vi "MM6.InitSpecDevs.vi"(0 "i ref in":refnum<vi>, 2 "InitObjs":string[](array[string]), 3 "ms timeout (10000)":i32=10000, 5 "error in (no error)":errorcluster) -> (14 "i ref out":refnum<vi>, 16 "InitObjs out":string[](array[string]), 17 "timed out":bool, 19 "error out":errorcluster)   [LabVIEW 2014, in "MM6.lvlib"]
doc: "Initializes the special devices"
uses:
  MM6.lvlib
  CS_Core/BaseProcess/BaseProcess.lvlib
  LEBITLib/LEBITLib.lvlib
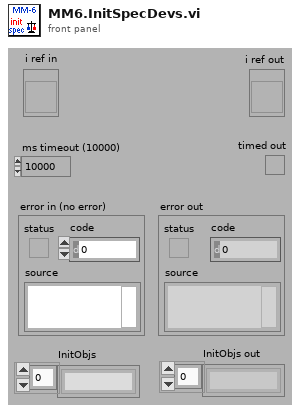
[diagram p1: front panel]
types:
  T1 = enum16{"simple", "synchronous", "asynchronous", "notification"}
  T2 = typedef "MM6.lvlib/MM6.i attribute.ctl" = cluster{"ConfigData":T3, "UsedObjs":string[], "ActScanStep":i32[], "AbortRequest":bool, "StopRequest":bool, "# cycles":i32, "Connected":bool, "MMStatus":T18, "# data":i32, "DIMServices":cluster{"MM6StatusString":string, "MM6StatusID":i32, "discArchiver":string, "discArchiverID":i32, "eventBuilder":string, "eventBuilderID":i32, "GUIIDString":string, "GUIIDStringID":i32}, "dataFile":string, "ExtraDataSets":T19, "PGRunning":T20}
  T3 = typedef "LEBITDefs.lvlib/LEBITDefs.ConfigData.ctl" = cluster{"GenConfig":T4, "Configs":T6[]}
  T4 = typedef "LEBITDefs.lvlib/LEBITDefs.GenConfig.ctl" = cluster{"Mode":i32, "Logs":T5[]}
  T5 = typedef "LEBITDefs.lvlib/LEBITDefs.Log.ctl" = cluster{"Name":string, "FctName":string, "Special":string}
  T6 = typedef "LEBITDefs.lvlib/LEBITDefs.OneConfig.ctl" = cluster{"MCA":T7, "Timing":T8, "Scans":T11[], "FreqDevs":T12[], "CleanDev":T13, "NrCycles":i32, "Specials":T15[], "Delays":T16[], "DAC":T17}
  T7 = typedef "LEBITDefs.lvlib/LEBITDefs.MCA.ctl" = cluster{"Name":string, "Address":string, "NrChannels":i32, "Gate":i32, "NrPipse":i32}
  T8 = typedef "LEBITDefs.lvlib/LEBITDefs.Timing.ctl" = cluster{"TimeTables":cluster{"TimeTable":T9}[], "Memories":T10[], "ScanX":string, "ScanY":string}
  T9 = typedef "LEBITDefs.lvlib/LEBITDefs.Timetable.ctl" = dbl[]
  T10 = typedef "LEBITDefs.lvlib/LEBITDefs.Memory.ctl" = cluster{"Device":string, "ExtTrig":bool, "TT2Use":i32, "PatternTable":string[]}
  T11 = typedef "LEBITDefs.lvlib/LEBITDefs.ScanDev.ctl" = cluster{"Name":string, "FctName":string, "Values":dbl[], "NrScanVals":i32, "Special":string}
  T12 = typedef "LEBITDefs.lvlib/LEBITDefs.FreqDev.ctl" = cluster{"Name":string, "Amp":dbl, "CenterFreq":dbl, "Time":dbl}
  T13 = typedef "LEBITDefs.lvlib/LEBITDefs.CleanDev.ctl" = cluster{"Name":string, "CleanData":T14[]}
  T14 = typedef "LEBITDefs.lvlib/LEBITDefs.CleanDataType.ctl" = cluster{"Amp":dbl, "Center":dbl, "Plus":dbl, "Minus":dbl, "Time":dbl}
  T15 = typedef "LEBITDefs.lvlib/LEBITDefs.Special.ctl" = cluster{"Name":string, "FctName":string, "VerySpecial":string, "Data":dbl}
  T16 = typedef "LEBITDefs.lvlib/LEBITDefs.Delay.ctl" = cluster{"Name":string, "Delay":dbl}
  T17 = typedef "LEBITDefs.lvlib/LEBITDefs.DAC.ctl" = cluster{"Name":string, "Step1":i32, "Step2":i32}
  T18 = typedef "MM6.lvlib/MM6.status.ctl" = enum16{"loaded", "load_error", "config", "config_error", "init", "init_error", "data_reset", "data_reset_error", "running", "start_error", "run_error", "abort_requested", "aborted", "stop_requested", "stopped", "stop_error", "Connected", "NOTConnected"}
  T19 = typedef "LEBITDefs.lvlib/LEBITDefs.ExtraData.ctl" = cluster{"Ions":cluster{"ExcitIonMass":string, "ExcitIonCharge":i32, "CleanIons":cluster{"CleanIonMass":string, "CleanIonCharge":i32}[]}, "TimingDescription":cluster{"TimeTableDescription":cluster{"Times":string[]}[], "PatternTableDescription":cluster{"Pattern":string[]}[]}, "ScanUnits":string[]}[]
  T20 = typedef "PPG_ABC.lvlib/PPG_ABC.PG_Running.ctl" = i32
  T21 = typedef "CoreDefs.rawDataType.ctl" = i8[]
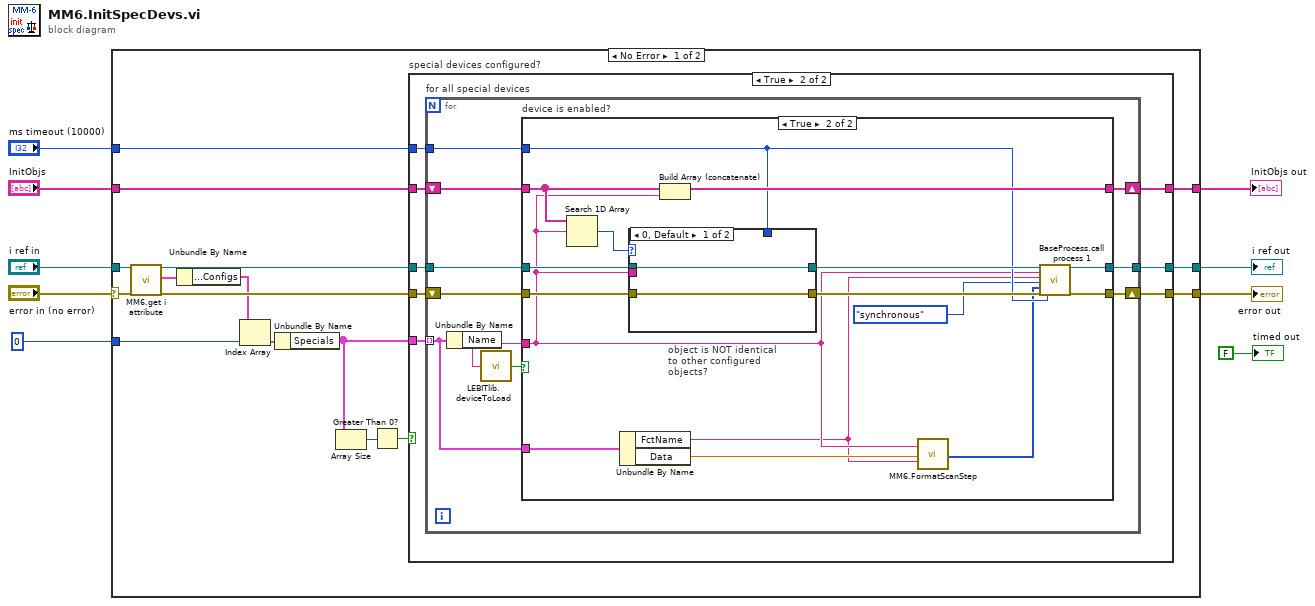
[diagram p0: block diagram]
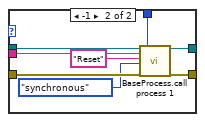
[diagram p4: hidden frame]
diagram:
  n1 = case shown="No Error" "error in (no error)" {
    selector: "error in (no error)" -> [w17 w76]
    tunnel: "i ref in" -> [w22 w77]
    tunnel: [w21 w77] -> w8
    tunnel: [w20 w76] -> w7
    tunnel: "InitObjs" -> [w19 w78]
    tunnel: [w18 w78] -> w4
    tunnel: 0 ("index") -> [w12 _]
    tunnel: "ms timeout (10000)" -> [w10 _]
    frame No Error {
      n2 = call "MM6.get i attribute.vi"("i ref in"=w22, "error in (no error)"=w17) -> ("i ref out"=w24:refnum<vi>, "i attribute"=w14:T2, "error out"=w23:errorcluster)  [unwired: 15 in]
      n3 = Unbundle By Name(w14) -> ("ConfigData.Configs"=w13:T6[])
      n4 = Index Array(array=w13, index=w12) -> (element=w11:T6)
      n5 = Unbundle By Name(w11) -> ("Specials"=w25:T15[])
      n6 = Array Size(array=w25) -> (size(s)=w15:i32)
      n7 = Greater Than 0?(x=w15) -> (x > 0?=w16:bool)
      n8 = case "special devices configured?" shown="True" w16 {
        tunnel: w25 -> [_ w36]
        tunnel: w24 -> [w28 w35]
        tunnel: [w28 w34] -> w21
        tunnel: w23 -> [w27 w30]
        tunnel: [w27 w31] -> w20
        tunnel: w19 -> [w26 w33]
        tunnel: [w26 w32] -> w18
        tunnel: w10 -> [_ w29]
        frame False {
        }
        frame True {
          n9 = for "for all special devices" {
            tunnel: w36 -> [w44] mode=indexing
            tunnel: w35 -> [w46]
            tunnel: [w45] -> w34
            shift-right: [w43] -> w32
            shift-left: w33 -> [w42]
            shift-right: [w41] -> w31
            shift-left: w30 -> [w40]
            tunnel: w29 -> [w37]
            n10 = Unbundle By Name(w44) -> ("Name"=w38:string)
            n11 = call "LEBITlib.deviceToLoad.vi"("DeviceName"=w38) -> ("DeviceIsToLoad"=w39:bool)
            n12 = case "device is enabled?" shown="True" w39 {
              tunnel: w46 -> [w49 w62]
              tunnel: [w49 w64] -> w45
              tunnel: w40 -> [w48 w61]
              tunnel: w38 -> [_ w51]
              tunnel: [w48 w63] -> w41
              tunnel: w44 -> [_ w65]
              tunnel: w42 -> [w47 w57]
              tunnel: [w47 w56] -> w43
              tunnel: w37 -> [_ w55]
              frame False {
              }
              frame True {
                n13 = Search 1D Array(1D array=w57, element=w51) -> (index of element=w58:i32)  [unwired: 1 in]
                n14 = Unbundle By Name(w65) -> ("FctName"=w50:string, "Data"=w52:dbl)
                n15 = case "object is NOT identical to other configured objects?" shown="0, Default" w58 {
                  tunnel: w62 -> [w67 w75]
                  tunnel: w61 -> [w66 w74]
                  tunnel: [w67 w73] -> w60
                  tunnel: [w66 w72] -> w59
                  tunnel: w51 -> [_ w71]
                  tunnel: w55 -> [_ w68]
                  frame 0, Default {
                  }
                  frame -1 {
                    n16 = call "BaseProcess.call process 1.vi"("i ref in"=w75, "Object"=w71, "Selector"="Reset", "CallType"=T1."synchronous", "error in (no error)"=w74, "timeout (ms)"=w68) -> ("i ref out"=w73:refnum<vi>, "error out"=w72:errorcluster)  [unwired: 11 in, 1 out]
                  }
                }
                n17 = Build Array (concatenate)(w57, w51) -> (w56:string[])
                n18 = call "MM6.FormatScanStep.vi"("Name"=w51, "Value"=w52, "FctName"=w50) -> ("byteArray out"=w53:T21)  [unwired: 15 in, 1 out]
                n19 = call "BaseProcess.call process 1.vi"("i ref in"=w60, "Object"=w51, "Selector"=w50, "CallType"=enum16{"simple", "synchronous", "asynchronous"}."synchronous", "Data"=w53, "error in (no error)"=w59, "timeout (ms)"=w55) -> ("i ref out"=w64:refnum<vi>, "error out"=w63:errorcluster)  [unwired: 10 in, 1 out]
              }
            }
          }
        }
      }
    }
    frame Error {
    }
  }
  "error out" <- w7
  "i ref out" <- w8
  "InitObjs out" <- w4
  "timed out" <- FALSE ("timed out")
